vi "Send mDNS Query.vi"(7 "timeout, ms (5000)":i32=5000, 8 "error in (no error)":errorcluster, 11 "query":T1 {"header"."opcode" items=["Query"=0, "IQuery"=1, "Status"=2, "Notify"=4, "Update"=5, "DSO"=6]; "questions"."class" items=["IN"=1, "CH"=3, "HS"=4, "NONE"=254, "*"=255]; "questions"."type" items=["A"=1, "NS"=2, "MD"=3, "MF"=4, "CNAME"=5, "SOA"=6, "MB"=7, "MG"=8, "MR"=9, "NULL"=10, "WKS"=11, "PTR"=12, "HINFO"=13, "MINFO"=14, "MX"=15, "TXT"=16, "RP"=17, "AFSDB"=18, "X25"=19, "ISDN"=20, "RT"=21, "NSAP"=22, "NSAP-PTR"=23, "SIG"=24, "KEY"=25, "PX"=26, "GPOS"=27, "AAAA"=28, "LOC"=29, "NXT"=30, "EID"=31, "NIMLOC"=32, "SRV"=33, "ATMA"=34, "NAPTR"=35, "KX"=36, "CERT"=37, "A6"=38, "DNAME"=39, "SINK"=40, "OPT"=41, "APL"=42, "DS"=43, "SSHFP"=44, "IPSECKEY"=45, "RRSIG"=46, "NSEC"=47, "DNSKEY"=48, "DHCID"=49, "NSEC3"=50, "NSEC3PARAM"=51, "TLSA"=52, "SMIMEA"=53, "HIP"=55, "NINFO"=56, "RKEY"=57, "TALINK"=58, "CDS"=59, "CDNSKEY"=60, "OPENPGPKEY"=61, "CSYNC"=62, "ZONEMD"=63, "SVCB"=64, "HTTPS"=65, "SPF"=99, "UINFO"=100, "UID"=101, "GID"=102, "UNSPEC"=103, "NID"=104, "L32"=105, "L64"=106, "LP"=107, "EUI48"=108, "EUI64"=109, "TKEY"=249, "TSIG"=250, "IXFR"=251, "AXFR"=252, "MAILB"=253, "MAILA"=254, "*"=255, "URI"=256, "CAA"=257, "AVC"=258, "DOA"=259, "AMTRELAY"=260, "TA"=32768, "DLV"=32769]}) -> (0 "error out":errorcluster, 2 "query id":u16, 3 "connection ID":refnum<k16>)   [LabVIEW 2015, in "PL DNS Client.lvlib"]
doc: "Sends Multicast DNS <b>query</b> and returns <b>connection ID</b> and <b>query id</b>."
uses:
  PL DNS Client.lvlib
  <vilib>/Utility/tcp.llb/UDP Multicast Read-Write Open.vi
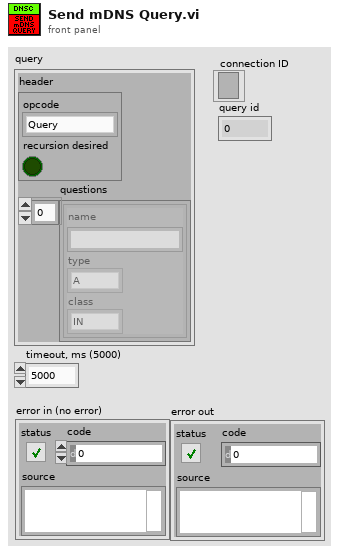
[diagram p1: front panel]
types:
  T1 = cluster{"header":cluster{"opcode":u8, "recursion desired":bool}, "questions":cluster{"name":string, "type":u16, "class":u16}[]}
  T2 = cluster{"name":string, "type":u16, "class":u16}[]
  T3 = cluster{u16, "opcode":u8, "recursion desired":bool}
  T4 = cluster{cluster{u16, "opcode":u8, "recursion desired":bool}, "questions":cluster{"name":string, "type":u16, "class":u16}[]}
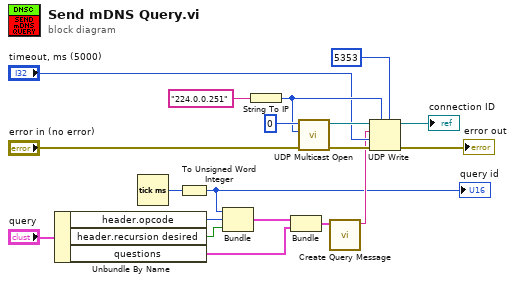
[diagram p0: block diagram]
diagram:
  n1 = Unbundle By Name("query") -> ("header.opcode"=w10:u8, "header.recursion desired"=w11:bool, "questions"=w6:T2)
  n2 = Tick Count (ms)() -> (millisecond timer value=w4:u32)
  n3 = To Unsigned Word Integer(number=w4) -> (unsigned 16bit integer=w3:u16)
  "query id" <- w3
  n4 = Bundle(w3, "opcode"=w10, "recursion desired"=w11) -> (w7:T3)  [unwired: 1 in]
  n5 = String To IP(1:"224.0.0.251" ("name")) -> (0:w16:u32)
  n6 = Bundle(w7, "questions"=w6) -> (w5:T4)  [unwired: 1 in]
  n7 = call-poly <vilib>:"UDP Multicast Open.vi"("error in (no error)"="error in (no error)", "multicast addr"=w16, "port"=u16 0) -> ("error out"=w18:errorcluster, "connection ID"=w17:refnum<k16>)  [unwired: 6 in, 1 out]
  n8 = call "Create Query Message.vi"("query"=w5) -> ("message"=w9:string)  [unwired: 10 in]
  n9 = UDP Write(address=w16, port or service name=u16 5353, connection ID=w17, data in=w9, 8:w18, 9:"timeout, ms (5000)") -> (error out=→"error out":errorcluster, 3:→"connection ID":refnum<k16>)
